vi "three_pitcher.vi"() -> ()   [LabVIEW 2021]
panel:
  out "result path":i32[][](array[numeric])
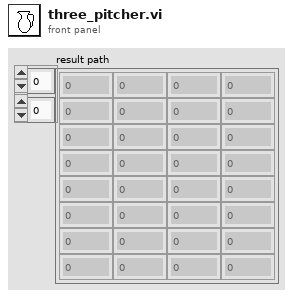
[diagram p1: front panel]
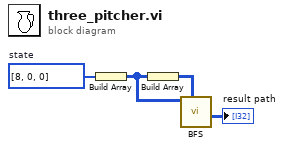
[diagram p0: block diagram]
diagram:
  w4 = i32[] [8, 0, 0]  # state
  n1 = Build Array(w4) -> (w2:i32[][])
  n2 = Build Array(w2) -> (w1:i32[][][])
  n3 = call "BFS.vi"("paths"=w1, "states"=w2) -> ("result path"=→"result path":i32[][])  [unwired: 9 in]
